vi "parse_twistWithCovariance.vi"(4 "error in":errorcluster, 7 "msg in":string) -> (0 "error out":errorcluster, 2 "TwistCovariance":T1, 3 "msg out":string)   [LabVIEW 2012]
doc: "Parses a message into a twist with covariance"
uses:
  <userlib>/ROS for LabVIEW Software/ROS/MessageParsing/std_msgs/subs/parse_float64_scalar.vi
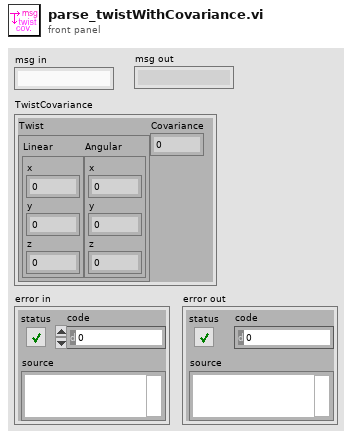
[diagram p1: front panel]
types:
  T1 = cluster{"Twist":cluster{"Linear":cluster{"x":dbl, "y":dbl, "z":dbl}, "Angular":cluster{"x":dbl, "y":dbl, "z":dbl}}, "Covariance":dbl}
  T2 = cluster{"Linear":cluster{"x":dbl, "y":dbl, "z":dbl}, "Angular":cluster{"x":dbl, "y":dbl, "z":dbl}}
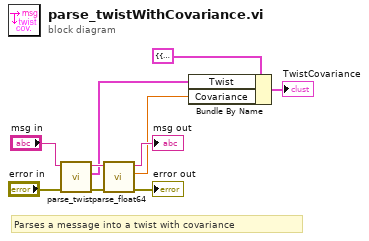
[diagram p0: block diagram]
diagram:
  # "Parses a message into a twist with covariance"
  n1 = call <userlib>:"parse_twist.vi"("error in"="error in", "msg in"="msg in") -> ("error out"=w7:errorcluster, "Twist"=w2:T2, "msg out"=w8:string)  [unwired: 3 in]
  n2 = call-poly <userlib>:"parse_float64.vi"("error in"=w7, "msg in"=w8) -> ("error out"=→"error out":errorcluster, "number"=w1:dbl, "msg out"=→"msg out":string)  [unwired: 3 in]
  n3 = Bundle By Name(cluster=T1 {"Twist"={"Linear"={"x"=0.0, "y"=0.0, "z"=0.0}, "Angular"={"x"=0.0, "y"=0.0, "z"=0.0}}, "Covariance"=0.0} ("TwistCovariance"), "Twist"=w2, "Covariance"=w1) -> (→"TwistCovariance":T1)
